vi "Transfer Command Handler.vi"(6 "Operator POVs":i16[](array[numeric]), 7 "Driver POVs":i16[](array[numeric]), 8 "Operator Axes":dbl[](array[numeric]), 9 "Operator Buttons":bool[](array[boolean]), 10 "Driver Buttons":bool[](array[boolean]), 11 "Driver Axes":dbl[](array[numeric])) -> ()   [LabVIEW 2019]
uses:
  4b2e57c4-e88b-492c-bc70-1c7325321079.vi
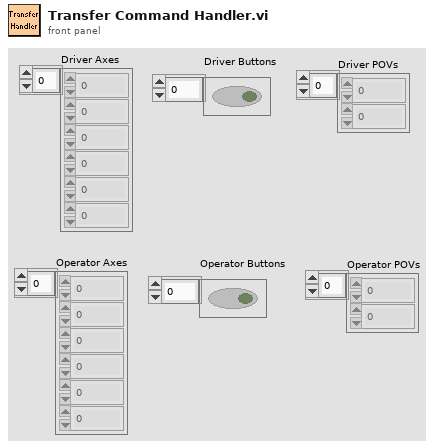
[diagram p1: front panel]
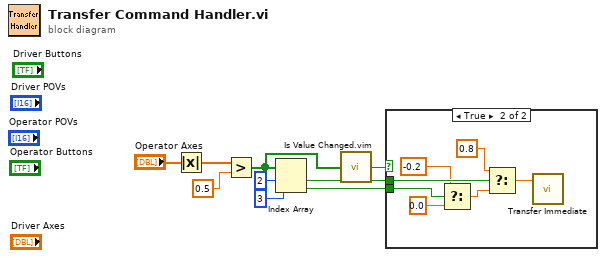
[diagram p0: block diagram]
diagram:
  n1 = Absolute Value(x="Operator Axes") -> (abs(x)=w1:dbl[])
  n2 = Greater?(x=w1, y=0.5) -> (0:w8:bool[])
  n3 = Index Array(array=w8, index #1=2 ("index"), index #2=3 ("index")) -> (element #1=w4:bool, element #2=w3:bool)
  n4 = call "Is Value Changed.vim"("value"=w8) -> ("changed or first call?"=w7:bool)
  n5 = case shown="True" w7 {
    tunnel: w4 -> [_ w16]
    tunnel: w3 -> [_ w13]
    frame False {
    }
    frame True {
      n6 = Select(t=-0.2, s=w13, f=0.0) -> (s? t:f=w14:dbl)
      n7 = Select(t=0.8, s=w16, f=w14) -> (s? t:f=w10:dbl)
      n8 = call "Transfer Immediate.vi"("Setpoint"=w10) -> ()  [unwired: 10 in, 1 out]
    }
  }
